vi "FPGAmain_5782_utan_AM.vi"() -> ()   [LabVIEW 2013]
uses:
  FPGA/DataMode.ctl
  FPGA/Input_5782/5782_states.ctl
  <vilib>/Platform/TimedLoop/XDataNode/timing_clust.ctl
  <vilib>/Platform/TimedLoop/XDataNode/nitl_modes.ctl
  <vilib>/Platform/TimedLoop/XDataNode/wakeup.ctl
  <vilib>/rvi/Emulation/niFpgaSctlEmulationGetInTimedLoop.vi
  <vilib>/rvi/Emulation/niFpgaEmulationReportErrorSimple.vi
  <vilib>/rvi/Emulation/niFpgaGetClockAttributes.vi
  <vilib>/rvi/eio/common/nirviEmuTemplateMethod_errors.vi
  <vilib>/rvi/Emulation/niFpgaCriticalErrorInLSC.vi
  <vilib>/rvi/FIFO/Fifo_Resource/nirvififoEmulationReadFpgaImpl.vi
  <vilib>/rvi/DataTransferAndStorage/Container/Common/niFpgaContainerGetUniqueNameForEmu.vi
  <vilib>/rvi/interface/RandomDataEmulation/nirviRandomDataFPGAFIFO.vi
  <vilib>/rvi/interface/RandomDataEmulation/niFpgaRandomDataHandleErrors.vi
  <vilib>/rvi/DataTransferAndStorage/Register/Emulation/niFpgaRegisterEmulationFpgaImpl.vi
  <instcachedir>/0/niFpgaRegisterEmulationFpgaImpl_DCF4BC0110594B98B44A971D60CEEC4D.lvgen/niFpgaRegisterEmulationFpgaImpl_DCF4BC0110594B98B44A971D60CEEC4D_003.vi
  <vilib>/rvi/FIFO/Fifo_Resource/nirvififoEmulationWriteFpgaImpl.vi
  <vilib>/Platform/TimedLoop/XDataNode/XDataNode.xnode
  <vilib>/eio/EIONode/EIONode.xnode
  <vilib>/rvi/DataTransferAndStorage/Container/XNode/niFpgaContainer.xnode
  <vilib>/rvi/FIFO/Fifo_Resource/nirvififoEmulationRead.vi
  <vilib>/rvi/interface/RandomDataEmulation/nirviRandomDataFpgaReadWriteTemplate.vi
  <vilib>/rvi/DataTransferAndStorage/Register/Emulation/niFpgaRegisterEmulation.vi
  <vilib>/rvi/FIFO/Fifo_Resource/nirvififoEmulationWrite.vi
  <vilib>/Platform/TimedLoop/XDataNode/XDNodeRunTimeDep.lvlib
panel:
  in  "b_am":fxp<+/-,16,2>
  in  "a_am":fxp<+/-,16,2>
  in  "AM phase":fxp<+,64,64>
  in  "DC offset chan 0":fxp<+/-,16,16>
  in  "DC offset chan 1":fxp<+/-,16,16>
  in  "delay phase":fxp<+,64,64>
  in  "User Command Commit":bool
  in  "User Command":u8
  out "User Command Idle":bool
  out "User Command Status":u8
  in  "User Data 0":u8
  in  "User Data 1":u8
  out "PLL Locked":bool
  out "User Error":bool
  out "Configured?":bool
  in  "Continuous":bool
  in  "trigger samples":u16=1
  in  "5782 record length":u16=4000 caption="Samples Per Trigger" min=1 step=1
  in  "Trigger Acquisition":bool
  out "IO Module\\Trigger Input":bool
  in  "quiet time":u16=4000
  in  "Downsample":fxp<+,8,8>=1.0
  in  "enable filter":bool
  in  "new coeffs":bool
  in  "FIR shift":i32
  in  "FIR coeffs":fxp<+/-,18,18>[](array[numeric])
  in  "Set downsample":bool
  in  "CIC Gain":fxp<+/-,32,1>=0.00390625 format="%#_32g"
  in  "Acquisition running":bool
  in  "Phase output":fxp<+,64,64>[](array[numeric])=[0.0, 0.0, 0.0, 0.0]
  in  "Simulated phase 5782":fxp<+,64,64>[](array[numeric])=[0.0, 0.0]
  in  "Mode":T1
  in  "Phase 5782":fxp<+,64,64>[](array[numeric])=[0.0, 0.0]
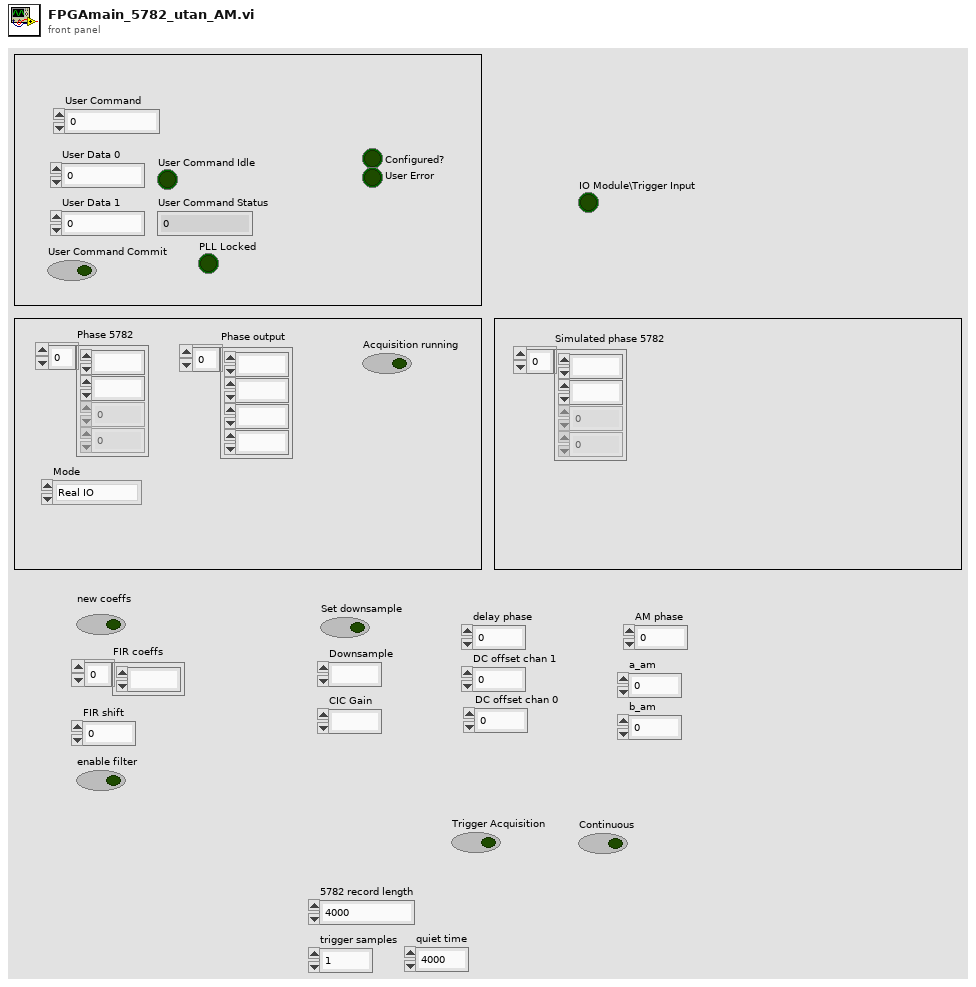
[diagram p1: front panel]
types:
  T1 = typedef "DataMode.ctl" = enum16{"Real IO", "Simulated"}
  T2 = typedef "5782_states.ctl" = enum8{"Wait for trigger", "Acquisition", "Send record length", "Quiet period"}
  T3 = typedef "XDNodeRunTimeDep.lvlib/timing_clust.ctl" = cluster{"Expected End [f-1]":u64, "Actual End [f-1]":u64, "Finished Late? [f-1]":bool, "Expected End [i-1]":u64, "Actual End [i-1]":u64, "Finished Late? [i-1]":bool, "Expected Start [i]":u64, "Actual Start [i]":u64, "Expected Start [f]":u64, "Actual Start [f]":u64, "Source Name":string, "Structure Name":string, "Period":i64, "Deadline":i64, "Offset":i64, "Start":i64, "Priority":i32, "Timeout":i32, "Mode":T4, "Wakeup Reason":T5, "Error":errorcluster, "Source Type":string, "Secondary Source Type":string, "Global End Time":u64, "Global Start Time":u64, "Frame Duration":u64, "Iteration Duration":u64, "Assigned CPU":i32, "I/O Scan Engine Mode":u32}
  T4 = typedef "XDNodeRunTimeDep.lvlib/nitl_modes.ctl" = enum32{"No Change", "Process missed periods, maintain original phase", "Discard missed periods, maintain original phase", "Process missed periods, ignore original phase", "Discard missed periods, ignore original phase"}
  T5 = typedef "XDNodeRunTimeDep.lvlib/wakeup.ctl" = enum32{"Normal", "Aborted", "Asynchronous wakeup", "Timing source error", "Timed loop error", "Timeout"}
  T6 = typedef "I16 array size 2.ctl" = i16[]
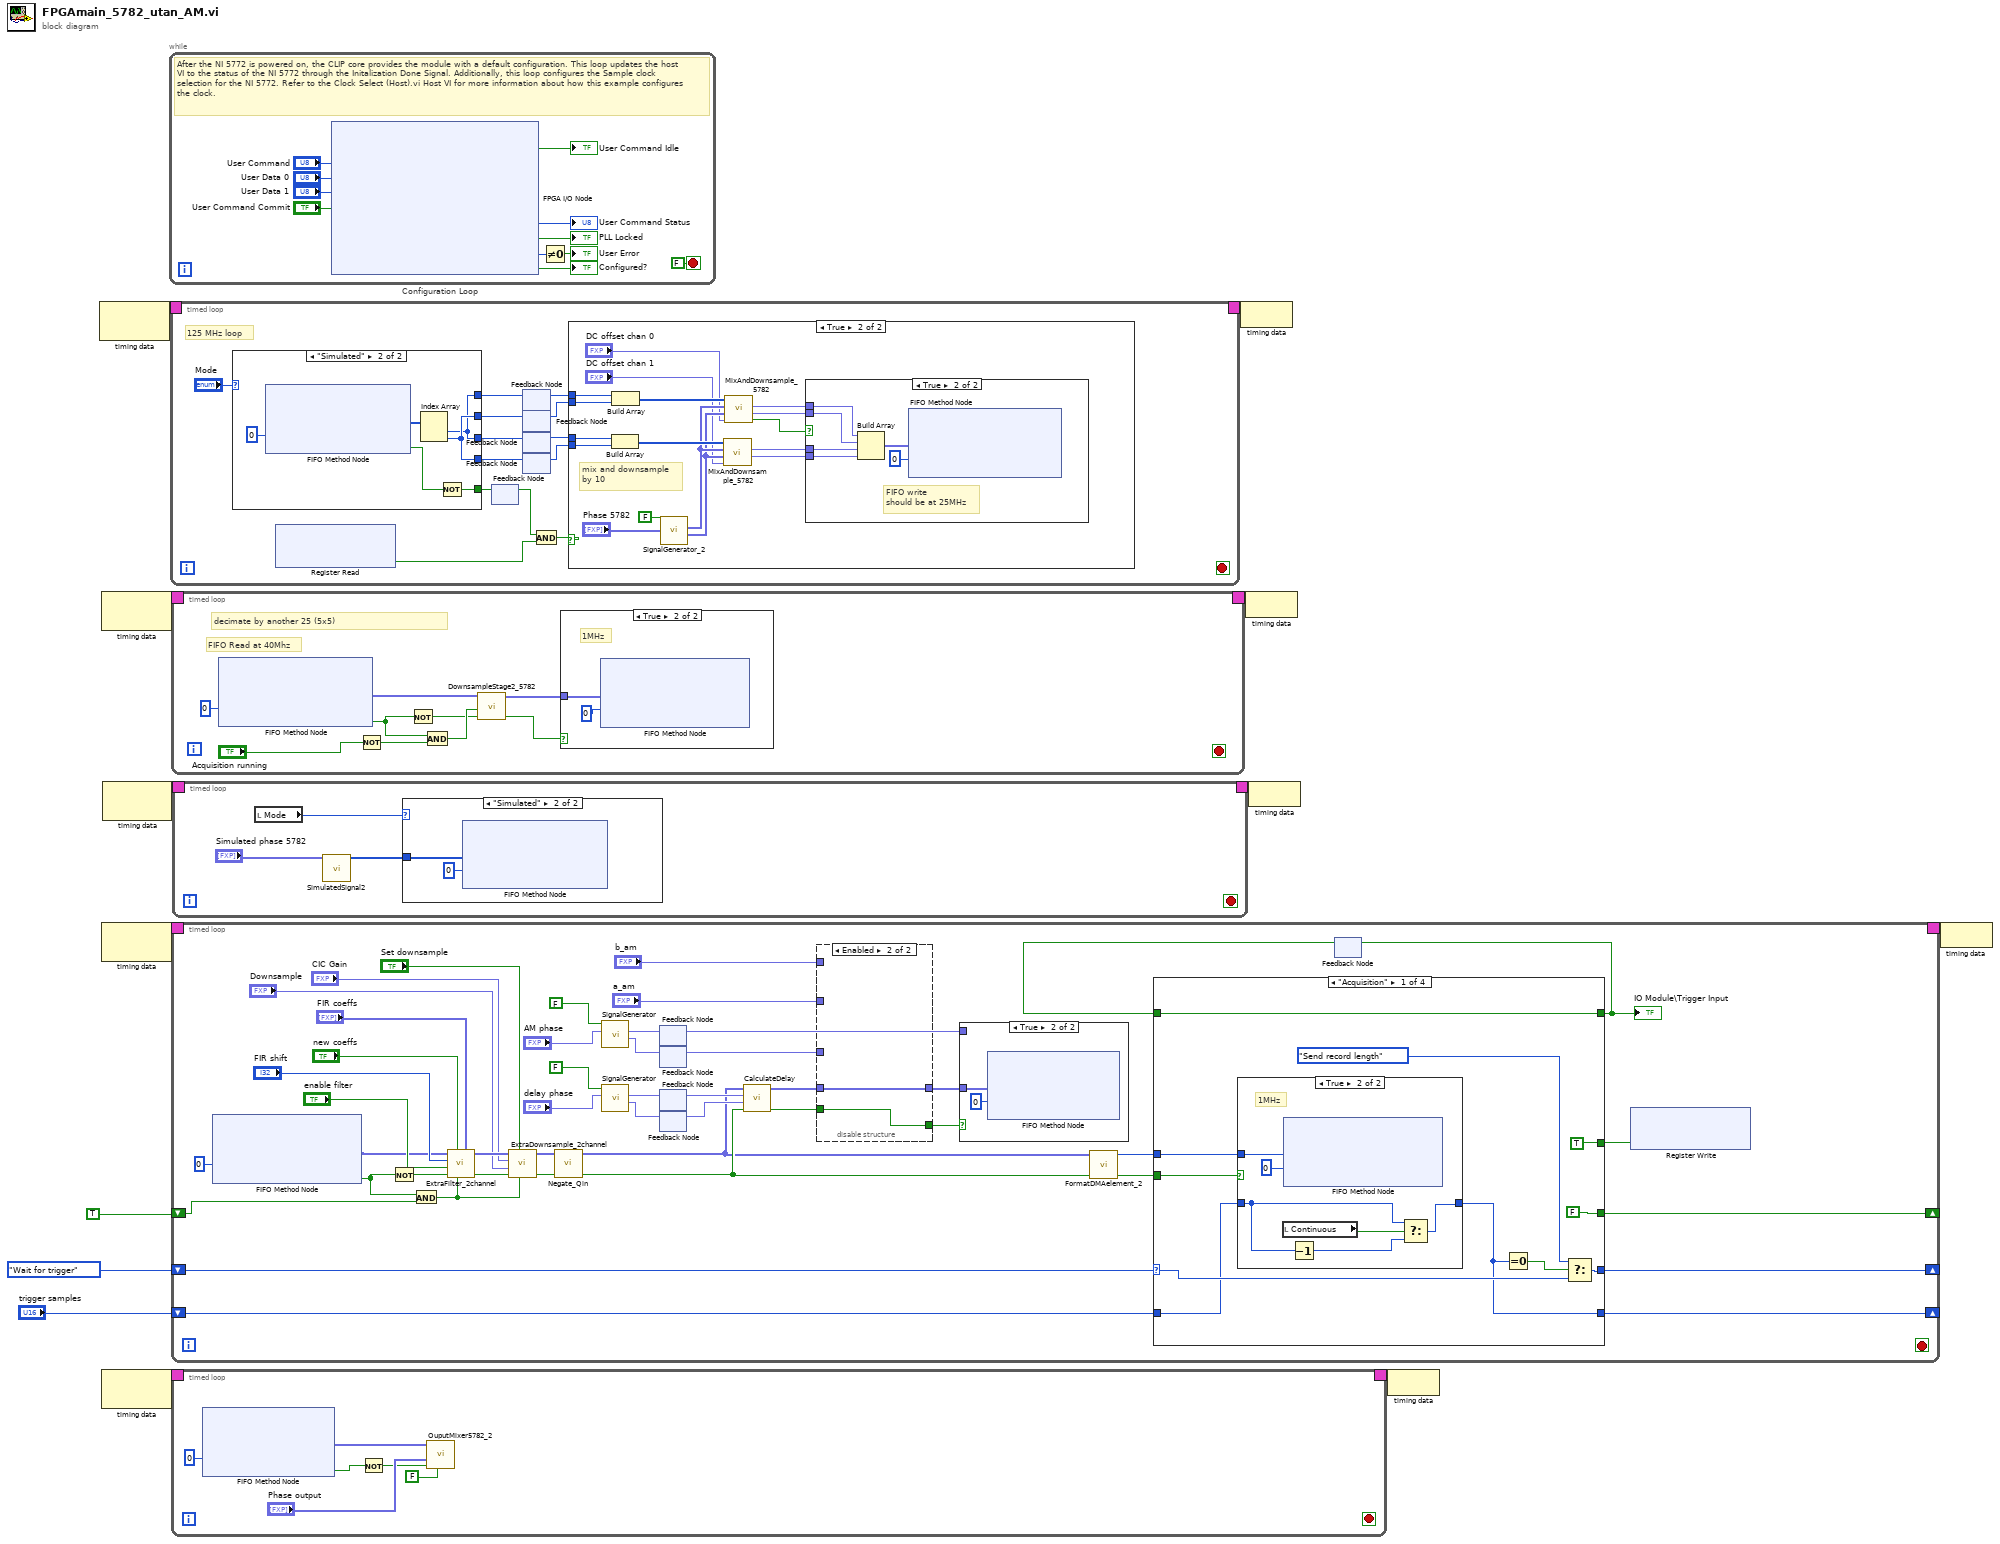
[diagram p0: block diagram]
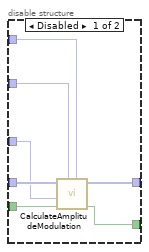
[diagram p2: hidden frame]
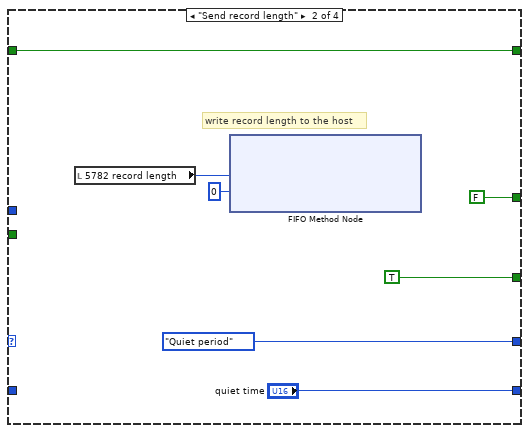
[diagram p5: hidden frame]
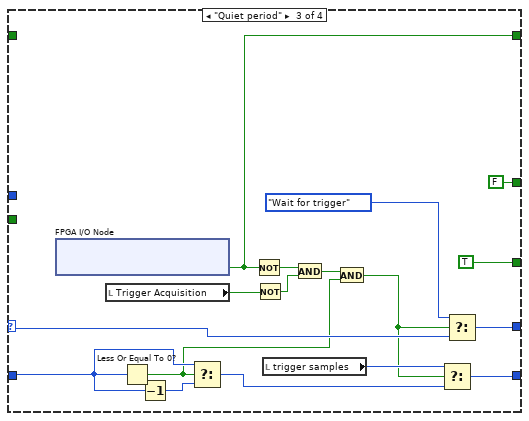
[diagram p6: hidden frame]
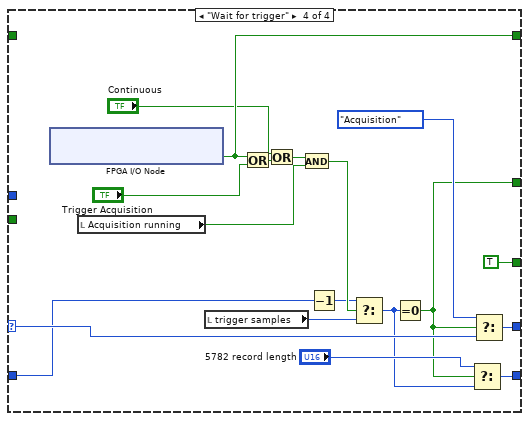
[diagram p7: hidden frame]
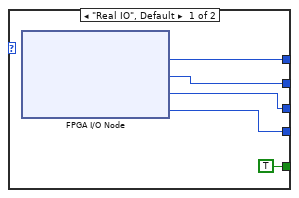
[diagram p10: hidden frame]
diagram:
  n1 = node-c288() -> (w9:T3)  [unwired: 1 in]
  n2 = node-c288() -> (w13:T3)  [unwired: 1 in]
  n3 = node-c288() -> (w7:T3)  [unwired: 1 in]
  n4 = node-c288() -> (w2:T3)  [unwired: 1 in]
  n5 = node-c288() -> (w11:T3)  [unwired: 1 in]
  n6 = while "Configuration Loop" {
    stop <- FALSE stop-if-true
    # "After the NI 5772 is powered on, the CLIP core provides the module with a default configuration. This loop updates the host VI to the status of the NI 5772 through the Initalization Done Signal. Additionally, this loop configures the Sample clock selection for the NI 5772. Refer to the Clock Select (Host).vi Host VI for more information about how this example configures the clock."
    n7 = xnode "FPGA I/O Node"("IO Module\\User Command"="User Command", "IO Module\\User Data 0"="User Data 0", "IO Module\\User Data 1"="User Data 1", "IO Module\\User Command Commit"="User Command Commit") -> ("IO Module\\User Command Idle"=→"User Command Idle":bool, "IO Module\\User Command Status"=→"User Command Status":u8, "IO Module\\PLL Locked"=→"PLL Locked":bool, "IO Module\\User Error"=w19:u8, "IO Module\\Initialization Done"=→"Configured?":bool)  [unwired: 9 in, 9 out]
    n8 = Not Equal To 0?(x=w19) -> (x != 0?=→"User Error":bool)
  }
  n9 = timed-loop {
    timing: w9 -> [_]
    timing-out: [_] -> w8
    stop <- _ stop-if-true
    # "125 MHz loop"
    n10 = case shown="\"Simulated\"" "Mode" {
      tunnel: [w65 w68] -> w35
      tunnel: [w64 w69] -> w33
      tunnel: [w63 w68] -> w31
      tunnel: [w62 w69] -> w28
      tunnel: [TRUE w66] -> w27
      frame "Real IO", Default {
        n11 = xnode "FPGA I/O Node"() -> ("IO Module\\AI 0 N-1"=w65:i16, "IO Module\\AI 0 N"=w64:i16, "IO Module\\AI 1 N-1"=w63:i16, "IO Module\\AI 1 N"=w62:i16)  [unwired: 4 in, 4 out]
      }
      frame "Simulated" {
        n12 = xnode ("FIFO Method Node")("Timeout"=0) -> ("Element"=w70:i16[], "Timed Out?"=w67:bool)  [unwired: 1 in, 1 out]
        n13 = Index Array(array=w70) -> (element #1=w68:i16, element #2=w69:i16)  [unwired: 2 in]
        n14 = Not(x=w67) -> (.not. x?=w66:bool)
      }
    }
    n15 = xnode ("Register Read")() -> ("Data"=w25:bool)  [unwired: 1 in, 1 out]
    n16 = feedback #1() -> (w26:bool)  [unwired: 1 in]
    n17 = feedback-in #1(w27) -> ()
    n18 = feedback #2() -> (w34:i16)  [unwired: 1 in]
    n19 = feedback-in #2(w35) -> ()
    n20 = feedback #3() -> (w32:i16)  [unwired: 1 in]
    n21 = feedback-in #3(w33) -> ()
    n22 = feedback #4() -> (w30:i16)  [unwired: 1 in]
    n23 = feedback-in #4(w31) -> ()
    n24 = feedback #5() -> (w29:i16)  [unwired: 1 in]
    n25 = feedback-in #5(w28) -> ()
    n26 = And(x=w26, y=w25) -> (x .and. y?=w36:bool)
    n27 = case shown="True" w36 {
      tunnel: w34 -> [_ w45]
      tunnel: w32 -> [_ w44]
      tunnel: w30 -> [_ w43]
      tunnel: w29 -> [_ w42]
      frame False {
      }
      frame True {
        # "mix and downsample\nby 10"
        n28 = Build Array(w43, w42) -> (w54:i16[])
        n29 = Build Array(w45, w44) -> (w41:i16[])
        n30 = call "SignalGenerator_2.vi"("Phase"="Phase 5782", "reset"=FALSE) -> ("Sine out"=w46:fxp<+/-,16,0>[], "Cosine out"=w47:fxp<+/-,16,0>[])  [unwired: 8 in]
        n31 = call "MixAndDownsample_5782.vi"("DC offset"="DC offset chan 1", "Sine in"=w46, "Cosine in"=w47, "Signal Input"=w54) -> ("Q out"=w49:fxp<+/-,16,14>, "I out"=w50:fxp<+/-,16,14>)  [unwired: 5 in, 1 out]
        n32 = call "MixAndDownsample_5782.vi"("DC offset"="DC offset chan 0", "Sine in"=w46, "Cosine in"=w47, "Signal Input"=w41) -> ("data valid"=w51:bool, "Q out"=w52:fxp<+/-,16,14>, "I out"=w53:fxp<+/-,16,14>)  [unwired: 5 in]
        n33 = case shown="True" w51 {
          tunnel: w52 -> [_ w60]
          tunnel: w53 -> [_ w57]
          tunnel: w50 -> [_ w56]
          tunnel: w49 -> [_ w55]
          frame False {
          }
          frame True {
            # "FIFO write\nshould be at 25MHz"
            n34 = Build Array(w57, w60, w56, w55) -> (w59:fxp<+/-,16,14>[])
            n35 = xnode ("FIFO Method Node")("Element"=w59, "Timeout"=0) -> ()  [unwired: 1 in, 2 out]
          }
        }
      }
    }
  }
  n36 = timed-loop {
    timing: w13 -> [_]
    timing-out: [_] -> w12
    stop <- _ stop-if-true
    # "FIFO Read at 40Mhz"
    # "decimate by another 25 (5x5)"
    n37 = xnode ("FIFO Method Node")("Timeout"=0) -> ("Element"=w81:fxp<+/-,16,14>[], "Timed Out?"=w77:bool)  [unwired: 1 in, 1 out]
    n38 = Not(x="Acquisition running") -> (.not. x?=w78:bool)
    n39 = Not(x=w77) -> (.not. x?=w75:bool)
    n40 = And(x=w77, y=w78) -> (x .and. y?=w76:bool)
    n41 = call "DownsampleStage2_5782.vi"("valid in"=w75, "reset"=w76, "Data in"=w81) -> ("valid out"=w79:bool, "data out"=w80:fxp<+/-,16,14>[])  [unwired: 7 in]
    n42 = case shown="True" w79 {
      tunnel: w80 -> [_ w83]
      frame False {
      }
      frame True {
        # "1MHz"
        n43 = xnode ("FIFO Method Node")("Element"=w83, "Timeout"=0) -> ()  [unwired: 1 in, 2 out]
      }
    }
  }
  n44 = timed-loop {
    timing: w7 -> [_]
    timing-out: [_] -> w6
    shift-right: [w131] -> _
    shift-left: 5782_states."Wait for trigger" ("5782 states") -> [w133]
    shift-right: [w130] -> _
    shift-left: "trigger samples" -> [w132]
    shift-right: [w112] -> _
    shift-left: TRUE -> [w115]
    stop <- _ stop-if-true
    n45 = xnode ("FIFO Method Node")("Timeout"=0) -> ("Element"=w117:fxp<+/-,16,14>[], "Timed Out?"=w116:bool)  [unwired: 1 in, 1 out]
    n46 = Not(x=w116) -> (.not. x?=w126:bool)
    n47 = And(x=w116, y=w115) -> (x .and. y?=w128:bool)
    n48 = call "ExtraFilter_2channel.vi"(5:"new coeffs"="FIR coeffs", "reset"=w128, 7:"new coeffs"="new coeffs", "valid in"=w126, "enable filter"="enable filter", "new shift"="FIR shift", "Data in"=w117) -> ("valid out"=w127:bool, "Data out"=w125:fxp<+/-,16,14>[])  [unwired: 3 in]
    n49 = call "ExtraDownsample_2channel.vi"("reset"=w128, "Set downsample"="Set downsample", "valid in"=w127, "Downsample"="Downsample", "CIC Gain"="CIC Gain", "Data in"=w125) -> ("valid out"=w107:bool, "Data out"=w108:fxp<+/-,16,14>[])  [unwired: 4 in]
    n50 = call "Negate_Qin.vi"("valid in"=w107, "Data in"=w108) -> ("valid out"=w88:bool, "Data out"=w87:fxp<+/-,16,14>[])  [unwired: 8 in]
    n51 = call "SignalGenerator.vi"("phase"="AM phase", "Reset"=FALSE) -> ("Cos"=w99:fxp<+/-,16,0>, "Sin"=w98:fxp<+/-,16,0>)  [unwired: 7 in, 1 out]
    n52 = call "SignalGenerator.vi"("phase"="delay phase", "Reset"=FALSE) -> ("Cos"=w103:fxp<+/-,16,0>, "Sin"=w104:fxp<+/-,16,0>)  [unwired: 7 in, 1 out]
    n53 = feedback #6() -> (w94:fxp<+/-,16,0>)  [unwired: 1 in]
    n54 = feedback-in #6(w98) -> ()
    n55 = feedback #7() -> (w95:fxp<+/-,16,0>)  [unwired: 1 in]
    n56 = feedback-in #7(w99) -> ()
    n57 = feedback-in #8(w104) -> ()
    n58 = feedback #8() -> (w102:fxp<+/-,16,0>)  [unwired: 1 in]
    n59 = feedback #9() -> (w101:fxp<+/-,16,0>)  [unwired: 1 in]
    n60 = feedback-in #9(w103) -> ()
    n61 = call "CalculateDelay.vi"("input valid"=w88, "cos_fi"=w101, "sin fi"=w102, "Data in"=w87) -> ("output valid"=w91:bool, "Data out"=w100:fxp<+/-,16,14>[])  [unwired: 6 in]
    n62 = disable-structure shown="Enabled" {
      disable-tunnel: w100 -> [w140 w142]
      disable-tunnel: w95 -> [w139 _]
      disable-tunnel: "a_am" -> [w138 _]
      disable-tunnel: "b_am" -> [w137 _]
      disable-tunnel: w91 -> [w136 w141]
      disable-tunnel: [w135 w142] -> w90
      disable-tunnel: [w134 w141] -> w89
      frame Disabled {
        n63 = call "CalculateAmplitudeModulation.vi"("b_am"=w137, "a_am"=w138, "input valid"=w136, "cos_am"=w139, "Data in"=w140) -> ("output valid"=w134:bool, "Data out"=w135:fxp<+/-,16,14>[])  [unwired: 5 in]
      }
      frame Enabled {
      }
    }
    n64 = case shown="True" w89 {
      tunnel: w90 -> [_ w143]
      tunnel: w94 -> [_ _]
      frame False {
      }
      frame True {
        n65 = xnode ("FIFO Method Node")("Element"=w143, "Timeout"=0) -> ()  [unwired: 1 in, 2 out]
      }
    }
    n66 = call "FormatDMAelement_2.vi"("valid in"=w88, "Data in"=w87) -> ("valid out"=w113:bool, "Element1"=w114:u64)  [unwired: 8 in]
    n67 = feedback #10() -> (w110:bool)  [unwired: 1 in]
    n68 = case shown="\"Acquisition\"" w133 {
      selector: w133 -> [w155 _ w184 w204]
      tunnel: w132 -> [w151 _ w172 w191]
      tunnel: [w154 5782_states."Quiet period" ("5782 states") w183 w203] -> w131
      tunnel: [w148 "quiet time" w186 w202] -> w130
      tunnel: w114 -> [w149 _ _ _]
      tunnel: w113 -> [w150 _ _ _]
      tunnel: [FALSE TRUE TRUE TRUE] -> w112
      tunnel: [TRUE FALSE ("5782 triggered") FALSE ("5782 triggered") w195] -> w111
      tunnel: [w147 w163 w174 w194] -> w109
      tunnel: w110 -> [w147 w163 _ _]
      frame "Acquisition" {
        n69 = case shown="True" w150 {
          tunnel: w149 -> [_ w162]
          tunnel: [w156 w159] -> w148
          tunnel: w151 -> [w156 w157]
          frame False {
          }
          frame True {
            # "1MHz"
            n70 = local read "Continuous"() -> (w160:bool)
            n71 = xnode ("FIFO Method Node")("Element"=w162, "Timeout"=0) -> ()  [unwired: 1 in, 2 out]
            n72 = Decrement(x=w157) -> (x-1=w158:u16)
            n73 = Select(t=w157, s=w160, f=w158) -> (s? t:f=w159:u16)
          }
        }
        n74 = Equal To 0?(x=w148) -> (x = 0?=w152:bool)
        n75 = Select(t=5782_states."Send record length" ("5782 states"), s=w152, f=w155) -> (s? t:f=w154:T2)
      }
      frame "Send record length" {
        # "write record length to the host"
        n76 = local read "5782 record length"() -> (w165:u16)
        n77 = xnode ("FIFO Method Node")("Element"=w165, "Timeout"=0) -> ()  [unwired: 1 in, 2 out]
      }
      frame "Quiet period" {
        n78 = xnode "FPGA I/O Node"() -> ("IO Module\\Trigger Input"=w174:bool)  [unwired: 1 in, 1 out]
        n79 = local read "Trigger Acquisition"() -> (w180:bool)
        n80 = Less Or Equal To 0?(x=w172) -> (x <= 0?=w171:bool)
        n81 = Decrement(x=w172) -> (x-1=w173:u16)
        n82 = Select(t=w172, s=w171, f=w173) -> (s? t:f=w170:u16)
        n83 = Not(x=w174) -> (.not. x?=w179:bool)
        n84 = Not(x=w180) -> (.not. x?=w178:bool)
        n85 = local read "trigger samples"() -> (w185:u16)
        n86 = And(x=w179, y=w178) -> (x .and. y?=w177:bool)
        n87 = And(x=w177, y=w171) -> (x .and. y?=w182:bool)
        n88 = Select(t=w185, s=w182, f=w170) -> (s? t:f=w186:u16)
        n89 = Select(t=5782_states."Wait for trigger" ("5782 states"), s=w182, f=w184) -> (s? t:f=w183:T2)
      }
      frame "Wait for trigger" {
        n90 = xnode "FPGA I/O Node"() -> ("IO Module\\Trigger Input"=w194:bool)  [unwired: 1 in, 1 out]
        n91 = local read "Acquisition running"() -> (w196:bool)
        n92 = local read "trigger samples"() -> (w190:u16)
        n93 = Or(x=w194, y="Trigger Acquisition") -> (x .or. y?=w189:bool)
        n94 = Or(x="Continuous", y=w189) -> (x .or. y?=w187:bool)
        n95 = And(x=w187, y=w196) -> (x .and. y?=w197:bool)
        n96 = Decrement(x=w191) -> (x-1=w192:u16)
        n97 = Select(t=w192, s=w197, f=w190) -> (s? t:f=w193:u16)
        n98 = Equal To 0?(x=w193) -> (x = 0?=w195:bool)
        n99 = Select(t="5782 record length", s=w195, f=w193) -> (s? t:f=w202:u16)
        n100 = Select(t=5782_states."Acquisition" ("5782 states"), s=w195, f=w204) -> (s? t:f=w203:T2)
      }
    }
    "IO Module\\Trigger Input" <- w109
    n101 = feedback-in #10(w109) -> ()
    n102 = xnode ("Register Write")("Data"=w111) -> ()  [unwired: 1 in, 1 out]
  }
  n103 = timed-loop {
    timing: w2 -> [_]
    timing-out: [_] -> w1
    stop <- _ stop-if-true
    n104 = xnode ("FIFO Method Node")("Timeout"=0) -> ("Element"=w209:fxp<+/-,16,14>[], "Timed Out?"=w211:bool)  [unwired: 1 in, 1 out]
    n105 = Not(x=w211) -> (.not. x?=w207:bool)
    n106 = call "OuputMixer5782_2.vi"("reset"=FALSE, "valid in"=w207, "Phase output"="Phase output", "Data in"=w209) -> ()  [unwired: 7 in, 1 out]
  }
  n107 = timed-loop {
    timing: w11 -> [_]
    timing-out: [_] -> w10
    stop <- _ stop-if-true
    n108 = local read "Mode"() -> (w217:T1)
    n109 = call "SimulatedSignal2.vi"("Phase"="Simulated phase 5782") -> ("output"=w216:T6)  [unwired: 9 in, 1 out]
    n110 = case shown="\"Simulated\"" w217 {
      tunnel: w216 -> [_ w218]
      frame "Real IO", Default {
      }
      frame "Simulated" {
        n111 = xnode ("FIFO Method Node")("Element"=w218, "Timeout"=0) -> ()  [unwired: 1 in, 2 out]
      }
    }
  }
  n112 = node-c288(w8) -> ()
  n113 = node-c288(w12) -> ()
  n114 = node-c288(w10) -> ()
  n115 = node-c288(w1) -> ()
  n116 = node-c288(w6) -> ()
